vi "re_call_plugin_lua.vi"(5 "LuaVIEW reference":T1) -> (15 "error out":errorcluster)   [LabVIEW 2012]
doc: "Opens a reference to a plug-in located at the specified path and calls that plug-in. When the path is relative, the plug-in will be searched for relative to the directory containing the calling task's main script. If the plug-in is not found there or if the calling script is not a task, the plug-in will be searched for relative to the resource base path. When running as a built application, the application executable will also be searched. When a VI with the specified name is already in memory, a reference to that VI is opened irrespective of the path.\n\nWhen the plug-in is not already in memory, it will be loaded unless the plug-in is a VI template, in which case an independent in-memory instance is created. Only when the plug-in is reentrant or a template is it possible to have simultaneous calls to different instances of the same plug-in implementation. The returned results are the same as those returned by the plug-in. On returning, the reference to the plug-in is closed which will cause its VI to be unloaded if no further references are open.\n\nPlug-ins typically implement protracted LabVIEW operations that must be startable and configurable from Lua. Plug-ins are referenced by path so that they can be located outside the built executable, which allows for adding, removal, or updating of plugins without the need of rebuilding and reinstalling the server. When multiple instances of the same plug-in must be simultaneously runnable, a template VI is usually preferable over a reentrant VI since template instances can have a unique front panel, can be individually debugged, and can remain running when calling an updated plug-in VI.\n\nTo configure a plug-in, provide a configuration table. The format of the table varies from plug-in to plug-in and typically reflects a LabVIEW cluster. When the plug-in does not require configuration, the table must be omitted. When the plug-in provides a default configuration, the entire table or named elements in the table can be omitted and will be substituted for by the default data.\nParameters:\nstr:path, path to the plug-in VI or template.\n[tab:config], optional configuration table to pass to the plug-in.\nResults:\n[any:result], result returned by plugin.\n...\nErrors:\nSpecified plug-in not found.\nConfiguration table is missing (when required by plug-in).\nConfiguration table has an invalid format.\nUnable to open plug-in VI reference.\nUnable to call plug-in, e.g. because its implementation is broken.\nAny errors returned by the plug-in being called."
uses:
  typedefs/t_LuaVIEW Reference.ctl
  subvis/private/LuaVIEW Pull (path).vi
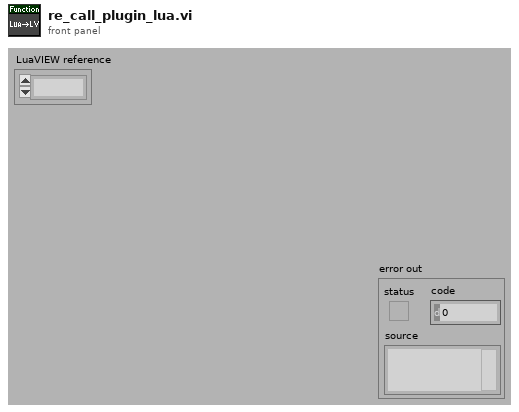
[diagram p1: front panel]
types:
  T1 = typedef "t_LuaVIEW Reference.ctl" = refnum<k1>
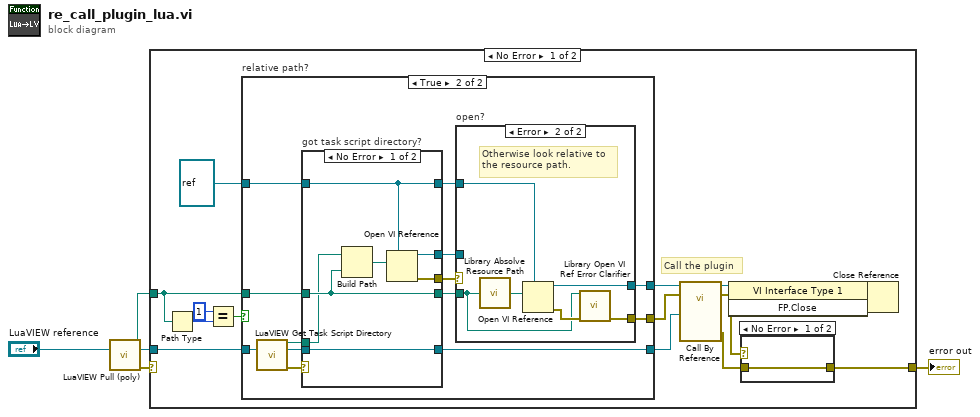
[diagram p0: block diagram]
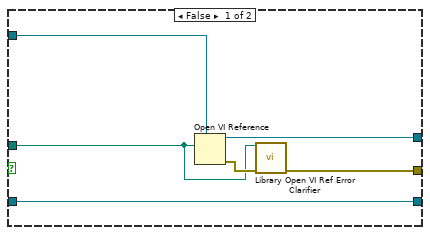
[diagram p2: hidden frame]
diagram:
  n1 = call-poly "LuaVIEW Pull (poly).vi"("LuaVIEW reference in"="LuaVIEW reference") -> ("path"=w4:path, "LuaVIEW reference out"=w2:T1, "error out"=w1:errorcluster)  [unwired: 12 in]
  n2 = case shown="No Error" w1 {
    selector: w1 -> [_ w60]
    tunnel: [w12 w60] -> w5
    tunnel: w4 -> [w9 _]
    tunnel: w2 -> [w14 _]
    frame No Error {
      # "Call the plugin"
      n3 = Path Type(1:w9) -> (0:w17:i16)
      n4 = Equal?(x=i16 1, y=w17) -> (x = y?=w15:bool)
      n5 = case "relative path?" shown="True" w15 {
        tunnel: w14 -> [w25 w29]
        tunnel: [w25 w36] -> w13
        tunnel: w9 -> [w23 w38]
        tunnel: [w22 w31] -> w7
        tunnel: [w21 w30] -> w8
        tunnel: refnum<vi> refnum ("plugin pane") -> [w20 w37]
        frame False {
          n6 = Open VI Reference(type specifier VI Refnum (for type only)=w20, vi path=w23) -> (vi reference=w21:refnum<vi>, error out=w24:errorcluster)  [unwired: 4 in]
          n7 = call "Library Open VI Ref Error Clarifier.vi"("VI path"=w23, "called VI error (no error)"=w24) -> ("error out"=w22:errorcluster)  [unwired: 13 in]
        }
        frame True {
          n8 = call "LuaVIEW Get Task Script Directory.vi"("LuaVIEW reference in"=w29) -> ("task script directory"=w27:path, "LuaVIEW reference out"=w28:T1, "error out"=w26:errorcluster)  [unwired: 12 in]
          n9 = case "got task script directory?" shown="No Error" w26 {
            selector: w26 -> [_ w54]
            tunnel: w38 -> [w51 w56]
            tunnel: w37 -> [w48 w55]
            tunnel: w28 -> [w52 w57]
            tunnel: [w52 w57] -> w36
            tunnel: [w51 w56] -> w33
            tunnel: [w50 w54] -> w35
            tunnel: [w49 _] -> w34
            tunnel: [w48 w55] -> w32
            tunnel: w27 -> [w47 _]
            frame No Error {
              n10 = Build Path(base path=w47, name or relative path=w51) -> (appended path=w53:path)
              n11 = Open VI Reference(type specifier VI Refnum (for type only)=w48, vi path=w53) -> (vi reference=w49:refnum<vi>, error out=w50:errorcluster)  [unwired: 4 in]
            }
            frame Error {
            }
          }
          n12 = case "open?" shown="Error" w35 {
            selector: w35 -> [w39 _]
            tunnel: w34 -> [w40 _]
            tunnel: w33 -> [_ w42]
            tunnel: w32 -> [_ w46]
            tunnel: [w39 w43] -> w31
            tunnel: [w40 w41] -> w30
            frame No Error {
            }
            frame Error {
              # "Otherwise look relative to\nthe resource path."
              n13 = call "Library Absolve Resource Path.vi"("path in"=w42) -> ("absolved path"=w45:path)  [unwired: 14 in]
              n14 = Open VI Reference(type specifier VI Refnum (for type only)=w46, vi path=w45) -> (vi reference=w41:refnum<vi>, error out=w44:errorcluster)  [unwired: 4 in]
              n15 = call "Library Open VI Ref Error Clarifier.vi"("VI path"=w42, "called VI error (no error)"=w44) -> ("error out"=w43:errorcluster)  [unwired: 13 in]
            }
          }
        }
      }
      n16 = call-by-ref "?"(reference=w8, error in=w7, "LuaVIEW reference"=w13) -> (reference out=w11:refnum<vi>, error out=w19:errorcluster, 15:"error out"=w18:errorcluster)  [unwired: 14 in]
      n17 = invoke class="VI Interface Type 1" method="FP.Close"(reference=w11) -> (reference out=w10:refnum<vi>)  [unwired: 2 in, 2 out]
      n18 = case shown="No Error" w19 {
        selector: w19 -> [_ w59]
        tunnel: [w58 w59] -> w12
        tunnel: w18 -> [w58 _]
        frame No Error {
        }
        frame Error {
        }
      }
      n19 = Close Reference(reference=w10) -> ()  [unwired: 1 in, 1 out]
    }
    frame Error {
    }
  }
  "error out" <- w5
